vi "_get_float4.vi"(7 "错误输入（无错误）":errorcluster, 8 "写入缓冲区":string, 9 "VISA资源名称":refnum<visa-resource-name>) -> (0 "错误输出":errorcluster, 1 "值 3":sgl, 2 "值 2":sgl, 3 "值":sgl, 4 "值 4":sgl, 5 "VISA资源名称输出":refnum<visa-resource-name>)   [LabVIEW 2017]
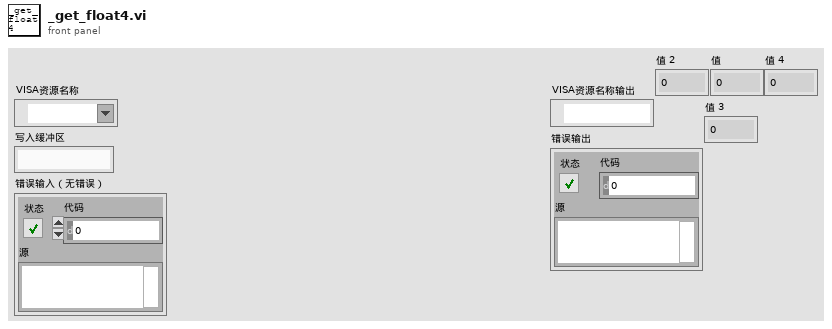
[diagram p1: front panel]
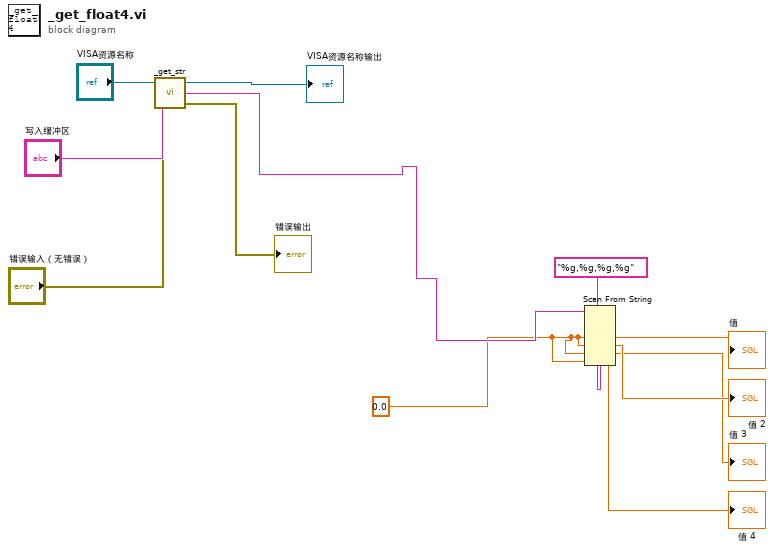
[diagram p0: block diagram]
diagram:
  w1 = sgl 0.0 ("默认值 1")
  n1 = call "_get_str.vi"("错误输入（无错误）"="错误输入（无错误）", "写入缓冲区"="写入缓冲区", "VISA资源名称"="VISA资源名称") -> ("错误输出"=→"错误输出":errorcluster, "读取缓冲区"=w7:string, "VISA资源名称输出"=→"VISA资源名称输出":refnum<visa-resource-name>)
  n2 = Scan From String(format string="%g,%g,%g,%g" ("格式字符串"), input string=w7, default 1=w1, default 2=w1, default 3=w1, default 4=w1) -> (output 1=→"值":sgl, output 2=→"值 2":sgl, output 3=→"值 3":sgl, output 4=→"值 4":sgl)  [unwired: 2 in, 3 out]
